vi "stopMotor.vi"(1 "ID":u32 format="%x", 2 "SPI Config In":T1) -> (0 "SPI Config Out":T1)   [LabVIEW 2019]
uses:
  SPI/SPI Config.ctl
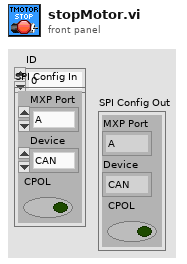
[diagram p1: front panel]
types:
  T1 = typedef "SPI Config.ctl" = cluster{"MXP Port":enum16{"A", "B"}, "Device":enum16{"CAN", "ENC", "IMU1", "IMU2"}, "CPOL":bool}
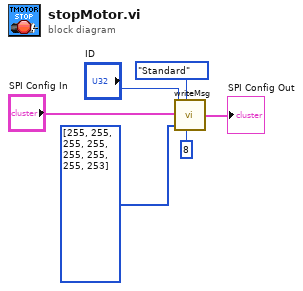
[diagram p0: block diagram]
diagram:
  n1 = call "writeMsg.vi"("ID"="ID", "ID Type"=enum16{"Standard", "Extended"}."Standard", "SPI Config In"="SPI Config In", "Data to Write"=u8[] [255, 255, 255, 255, 255, 255, 255, 253], "Frames to Write"=u8 8) -> ("SPI Config Out"=→"SPI Config Out":T1)
